vi "JSON GENERADOR PARAMETROS.vi"(5 "enige_hours":sgl, 7 "power_gen":dbl, 8 "error in":errorcluster, 9 "power_factor":dbl, 10 "fuel_usage":dbl, 11 "time":u32) -> (0 "error out":errorcluster, 3 "JSON Object out":refnum<class "JSON Object.lvclass">)   [LabVIEW 2015]
uses:
  <vilib>/addons/JSON API/Get Polymorphic/JSON GetSet.lvlib
  <vilib>/addons/JSON API/JSON Scalar/Set SGL.vi
  <vilib>/addons/JSON API/JSON Scalar/JSON Scalar.lvclass
  <vilib>/addons/JSON API/JSON Object/Set Object Item by name.vi
  <vilib>/addons/JSON API/JSON Object/JSON Object.lvclass
  <vilib>/addons/JSON API/JSON Scalar/Set DBL.vi
  <vilib>/addons/JSON API/JSON Scalar/Set U32.vi
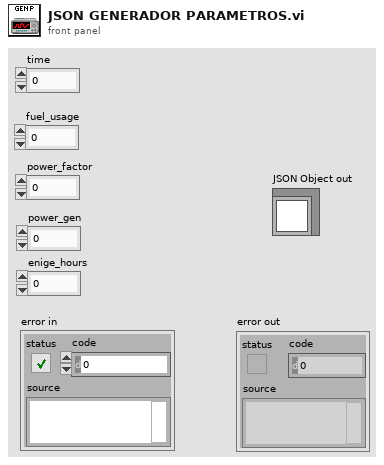
[diagram p1: front panel]
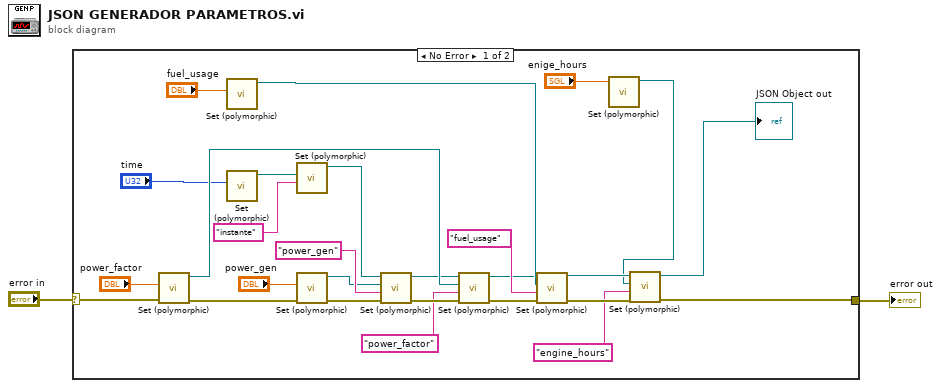
[diagram p0: block diagram]
diagram:
  n1 = case shown="No Error" "error in" {
    selector: "error in" -> [w10 w30]
    tunnel: [w3 w30] -> w2
    frame No Error {
      n2 = call-poly <vilib>:"Set (polymorphic).vi"("error in (no error)"=w10, "Numeric"="power_factor") -> ("error out"=w11:errorcluster, "JSON Scalar out"=w24:refnum<class "JSON Scalar.lvclass">)  [unwired: 8 in]
      n3 = call-poly <vilib>:"Set (polymorphic).vi"("Numeric"="fuel_usage") -> ("JSON Scalar out"=w27:refnum<class "JSON Scalar.lvclass">)  [unwired: 9 in, 1 out]
      n4 = call-poly <vilib>:"Set (polymorphic).vi"("Numeric"="time") -> ("JSON Scalar out"=w14:refnum<class "JSON Scalar.lvclass">)  [unwired: 9 in, 1 out]
      n5 = call-poly <vilib>:"Set (polymorphic).vi"("name"="instante", "Value"=w14) -> ("JSON Object out"=w12:refnum<class "JSON Object.lvclass">)  [unwired: 7 in, 2 out]
      n6 = call-poly <vilib>:"Set (polymorphic).vi"("error in (no error)"=w11, "Numeric"="power_gen") -> ("error out"=w20:errorcluster, "JSON Scalar out"=w18:refnum<class "JSON Scalar.lvclass">)  [unwired: 8 in]
      n7 = call-poly <vilib>:"Set (polymorphic).vi"("error in (no error)"=w20, "name"="power_gen", "Value"=w18, "JSON Object in"=w12) -> ("error out"=w23:errorcluster, "JSON Object out"=w21:refnum<class "JSON Object.lvclass">)  [unwired: 5 in, 1 out]
      n8 = call-poly <vilib>:"Set (polymorphic).vi"("error in (no error)"=w23, "name"="power_factor", "Value"=w24, "JSON Object in"=w21) -> ("error out"=w29:errorcluster, "JSON Object out"=w25:refnum<class "JSON Object.lvclass">)  [unwired: 5 in, 1 out]
      n9 = call-poly <vilib>:"Set (polymorphic).vi"("error in (no error)"=w29, "name"="fuel_usage", "Value"=w27, "JSON Object in"=w25) -> ("error out"=w9:errorcluster, "JSON Object out"=w8:refnum<class "JSON Object.lvclass">)  [unwired: 5 in, 1 out]
      n10 = call-poly <vilib>:"Set (polymorphic).vi"("Numeric"="enige_hours") -> ("JSON Scalar out"=w5:refnum<class "JSON Scalar.lvclass">)  [unwired: 9 in, 1 out]
      n11 = call-poly <vilib>:"Set (polymorphic).vi"("error in (no error)"=w9, "name"="engine_hours", "Value"=w5, "JSON Object in"=w8) -> ("error out"=w3:errorcluster, "JSON Object out"=→"JSON Object out":refnum<class "JSON Object.lvclass">)  [unwired: 5 in, 1 out]
    }
    frame Error {
    }
  }
  "error out" <- w2
